vi "ep_Error Checking.vi"(7 "reset? (F)":bool, 8 "error in (no error)":errorcluster, 9 "filter for frequency measurement":T1={"enable filter? (T)"=TRUE, "passband edge frequency [Hz]"=0.0, "passband ripple [dB]"=0.1, "stopband edge frequency [Hz]"=0.0, "stopband attenuation [dB]"=60.0}, 10 "frequency range [Hz]":cluster{"minimum":dbl, "maximum":dbl}, 11 "reference signal":waveform(dbl)) -> (0 "error out":errorcluster, 1 "dup filter for frequency measurement":T1={"enable filter? (T)"=TRUE, "passband edge frequency [Hz]"=0.0, "passband ripple [dB]"=0.1, "stopband edge frequency [Hz]"=0.0, "stopband attenuation [dB]"=60.0}, 2 "dup frequency range [Hz]":cluster{"minimum":dbl, "maximum":dbl}, 3 "dup reference signal":waveform(dbl))   [LabVIEW 2013, in "NI_EP_Power Measurement.lvlib"]
uses:
  <vilib>/addons/Electrical Power/Power Measurement/NI_EP_Power Measurement.lvlib
  <vilib>/addons/Electrical Power/Power Measurement/subVIs/ep_Filter Design.ctl
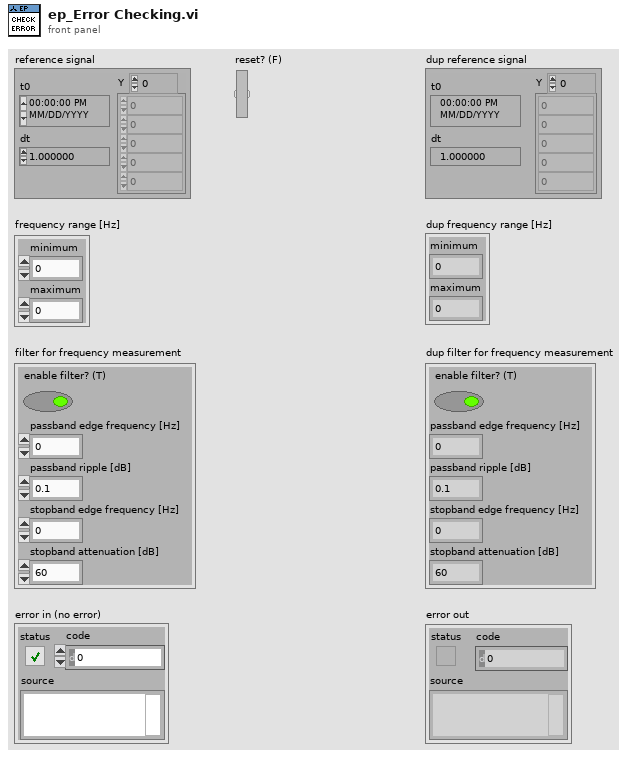
[diagram p1: front panel]
types:
  T1 = typedef "NI_EP_Power Measurement.lvlib/ep_Filter Design.ctl" = cluster{"enable filter? (T)":bool, "passband edge frequency [Hz]":dbl, "passband ripple [dB]":dbl, "stopband edge frequency [Hz]":dbl, "stopband attenuation [dB]":dbl}
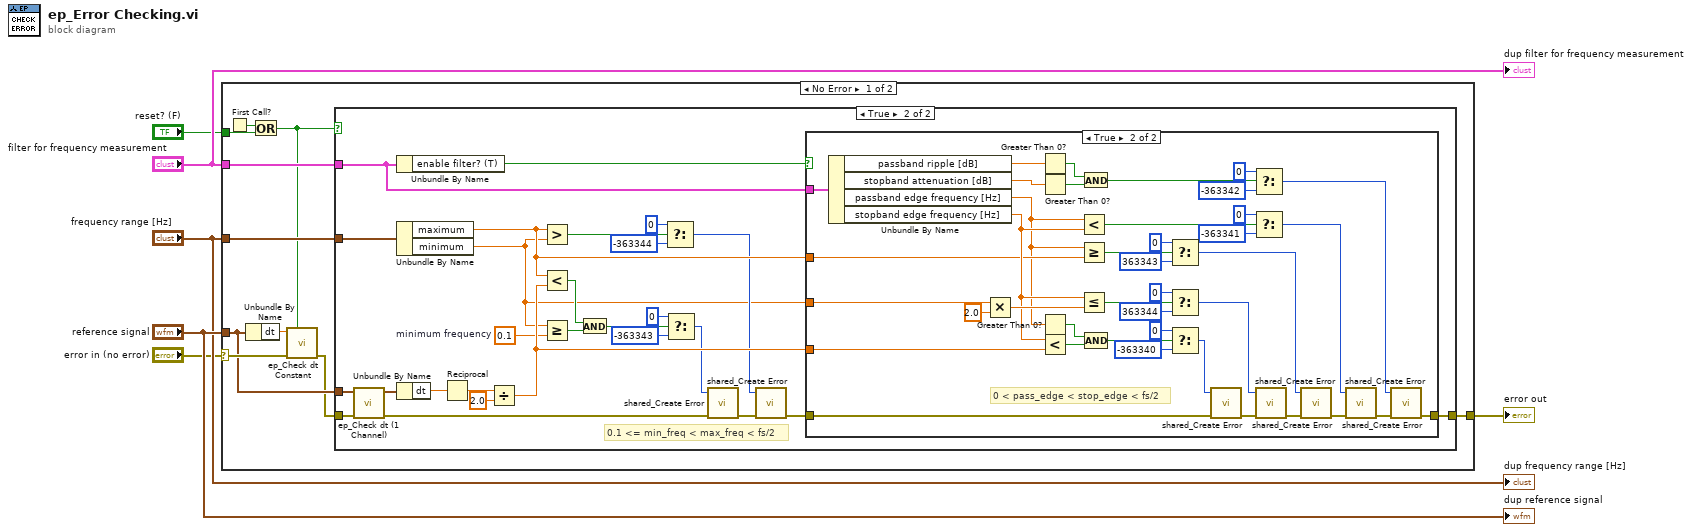
[diagram p0: block diagram]
diagram:
  n1 = case shown="No Error" "error in (no error)" {
    selector: "error in (no error)" -> [w11 w86]
    tunnel: "reference signal" -> [w8 _]
    tunnel: "filter for frequency measurement" -> [w15 _]
    tunnel: "frequency range [Hz]" -> [w14 _]
    tunnel: [w16 w86] -> w3
    tunnel: "reset? (F)" -> [w13 _]
    frame No Error {
      n2 = First Call?() -> (First Call?: T/F=w12:bool)
      n3 = Unbundle By Name(w8) -> ("dt"=w9:dbl)
      n4 = Or(x=w12, y=w13) -> (x .or. y?=w10:bool)
      n5 = call <vilib>:"ep_Check dt Constant.vi"("reset? (F)"=w10, "error in (no error)"=w11, "dt"=w9) -> ("error out"=w7:errorcluster)  [unwired: 7 in, 1 out]
      n6 = case shown="True" w10 {
        tunnel: w8 -> [_ w25]
        tunnel: w7 -> [w17 w26]
        tunnel: [w17 w37] -> w16
        tunnel: w14 -> [_ w33]
        tunnel: w15 -> [_ w32]
        frame False {
        }
        frame True {
          w18 = 0.1  # minimum frequency
          # "0.1 <= min_freq < max_freq < fs/2"
          n7 = call <vilib>:"ep_Check dt (1 Channel).vi"("error in (no error)"=w26, "waveform in"=w25) -> ("error out"=w27:errorcluster, "waveform out"=w24:waveform(dbl))  [unwired: 8 in]
          n8 = Unbundle By Name(w32) -> ("enable filter? (T)"=w38:bool)
          n9 = Unbundle By Name(w33) -> ("maximum"=w31:dbl, "minimum"=w19:dbl)
          n10 = Unbundle By Name(w24) -> ("dt"=w36:dbl)
          n11 = Reciprocal(x=w36) -> (1/x=w35:dbl)
          n12 = Divide(x=w35, y=2.0) -> (x/y=w30:dbl)
          n13 = Greater?(x=w31, y=w19) -> (0:w44:bool)
          n14 = Less?(x=w31, y=w30) -> (x < y?=w21:bool)
          n15 = Greater Or Equal?(x=w19, y=w18) -> (x >= y?=w22:bool)
          n16 = And(x=w21, y=w22) -> (x .and. y?=w20:bool)
          n17 = Select(t=0 ("error code (0)"), s=w44, f=-363344 ("error code (0)")) -> (s? t:f=w28:i32)
          n18 = Select(t=0 ("error code (0)"), s=w20, f=-363343 ("error code (0)")) -> (s? t:f=w29:i32)
          n19 = call <vilib>:"shared_Create Error.vi"("error in (no error)"=w27, "error code (0)"=w29) -> ("error out"=w23:errorcluster)  [unwired: 9 in]
          n20 = call <vilib>:"shared_Create Error.vi"("error in (no error)"=w23, "error code (0)"=w28) -> ("error out"=w39:errorcluster)  [unwired: 9 in]
          n21 = case shown="True" w38 {
            tunnel: w39 -> [w45 w59]
            tunnel: w32 -> [_ w72]
            tunnel: [w45 w52] -> w37
            tunnel: w30 -> [_ w47]
            tunnel: w31 -> [_ w67]
            tunnel: w19 -> [_ w71]
            frame False {
            }
            frame True {
              # "0 < pass_edge < stop_edge < fs/2"
              n22 = Unbundle By Name(w72) -> ("passband ripple [dB]"=w85:dbl, "stopband attenuation [dB]"=w79:dbl, "passband edge frequency [Hz]"=w66:dbl, "stopband edge frequency [Hz]"=w68:dbl)
              n23 = Multiply(x=w71, y=2.0) -> (x*y=w69:dbl)
              n24 = Greater Than 0?(x=w85) -> (x > 0?=w83:bool)
              n25 = Greater Than 0?(x=w79) -> (x > 0?=w84:bool)
              n26 = Greater Than 0?(x=w66) -> (x > 0?=w48:bool)
              n27 = Less?(x=w68, y=w47) -> (x < y?=w46:bool)
              n28 = Less?(x=w66, y=w68) -> (x < y?=w73:bool)
              n29 = Greater Or Equal?(x=w66, y=w67) -> (x >= y?=w63:bool)
              n30 = Less Or Equal?(x=w68, y=w69) -> (x <= y?=w60:bool)
              n31 = And(x=w83, y=w84) -> (x .and. y?=w82:bool)
              n32 = Compound Arithmetic op=AND(w48, w46) -> (w76:bool)
              n33 = Select(t=0 ("error code (0)"), s=w63, f=363343 ("error code (0)")) -> (s? t:f=w51:i32)
              n34 = Select(t=0 ("error code (0)"), s=w60, f=363344 ("error code (0)")) -> (s? t:f=w56:i32)
              n35 = Select(t=0 ("error code (0)"), s=w76, f=-363340 ("error code (0)")) -> (s? t:f=w58:i32)
              n36 = call <vilib>:"shared_Create Error.vi"("error in (no error)"=w59, "error code (0)"=w58) -> ("error out"=w57:errorcluster)  [unwired: 9 in]
              n37 = Select(t=0 ("error code (0)"), s=w82, f=-363342 ("error code (0)")) -> (s? t:f=w49:i32)
              n38 = Select(t=0 ("error code (0)"), s=w73, f=-363341 ("error code (0)")) -> (s? t:f=w50:i32)
              n39 = call <vilib>:"shared_Create Error.vi"("error in (no error)"=w57, "error code (0)"=w56) -> ("error out"=w55:errorcluster)  [unwired: 9 in]
              n40 = call <vilib>:"shared_Create Error.vi"("error in (no error)"=w55, "error code (0)"=w51) -> ("error out"=w54:errorcluster)  [unwired: 9 in]
              n41 = call <vilib>:"shared_Create Error.vi"("error in (no error)"=w54, "error code (0)"=w50) -> ("error out"=w53:errorcluster)  [unwired: 9 in]
              n42 = call <vilib>:"shared_Create Error.vi"("error in (no error)"=w53, "error code (0)"=w49) -> ("error out"=w52:errorcluster)  [unwired: 9 in]
            }
          }
        }
      }
    }
    frame Error {
    }
  }
  "error out" <- w3
  "dup frequency range [Hz]" <- "frequency range [Hz]"
  "dup reference signal" <- "reference signal"
  "dup filter for frequency measurement" <- "filter for frequency measurement"
